vi "Send Command Response.vi"(0 "LVx - Template Command in":refnum<class "REx - NART - Unoad DUT.lvclass">, 11 "error in (no error)":errorcluster) -> (4 "LVx - Template Command out":refnum<class "REx - NART - Unoad DUT.lvclass">, 15 "error out":errorcluster)   [LabVIEW 2011, in "ART2 Test Panel.lvlib" / "REx - NART - Unoad DUT.lvclass"]
uses:
  REx - NART - Unoad DUT.lvclass
  LVx Folder/LVx.lvclass
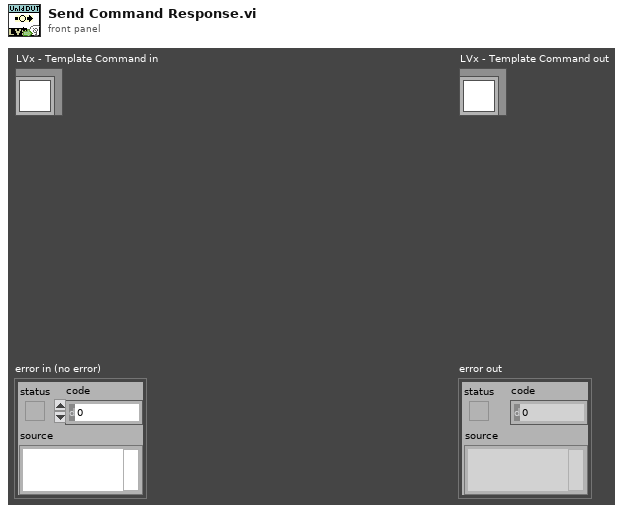
[diagram p1: front panel]
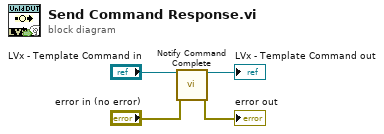
[diagram p0: block diagram]
diagram:
  n1 = call "Notify Command Complete.vi"("LVx.lvlib:LVx.lvclass"="LVx - Template Command in", "error in (no error)"="error in (no error)") -> ("LVx.lvclass out"=→"LVx - Template Command out":refnum<class "REx - NART - Unoad DUT.lvclass">, "error out"=→"error out":errorcluster)  [unwired: 12 in]
